vi "LVClass_Pupil AND operator.vi"(0 "Pupil A in":refnum<class "Pupil.lvclass">, 5 "Pupil B":refnum<class "Pupil.lvclass">, 11 "error in (no error)":errorcluster) -> (4 "Pupil A out":refnum<class "Pupil.lvclass">, 15 "error out":errorcluster)   [LabVIEW 2020, in "Pupil.lvclass"]
doc: "Pupil assignment.\n\n--------------------------------------------------------------------------------\n\n<B>Pupil_dstIn </B> : Pupil object.\n<B>Pupil_dstOut </B> : Pupil object.\n<B>Pupil_src </B> : Pupil object to copy.\n<B>ErrorIn </B> : Error\n<B>ErrorOut </B> : Error\n\n--------------------------------------------------------------------------------"
uses:
  Pupil.lvclass
  Pupil.lvclass/Pupil.ctl
  LVClass_Pupil Read Pupil.vi
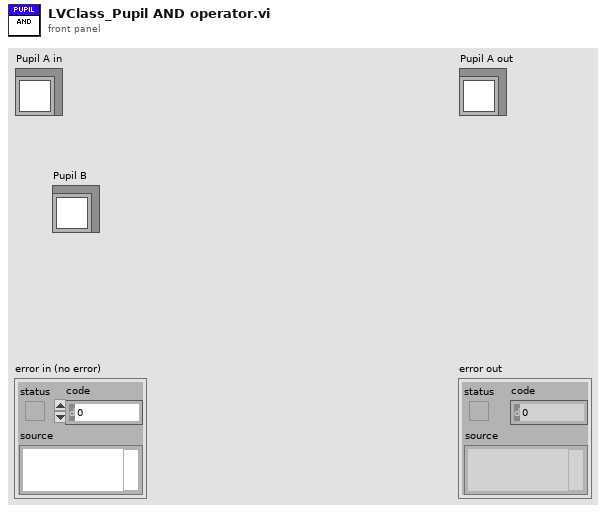
[diagram p1: front panel]
types:
  T1 = typedef "ClassID.ctl" = i64
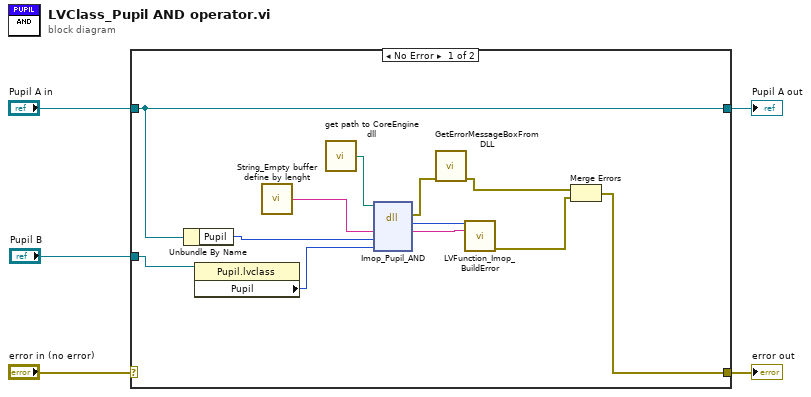
[diagram p0: block diagram]
diagram:
  n1 = case shown="No Error" "error in (no error)" {
    selector: "error in (no error)" -> [_ w19]
    tunnel: [w6 w19] -> w5
    tunnel: [w12 w18] -> w4
    tunnel: "Pupil A in" -> [w12 w18]
    tunnel: "Pupil B" -> [w10 _]
    frame No Error {
      n2 = Unbundle By Name(w12) -> ("Pupil"=w11:T1)
      n3 = property class="Pupil.lvclass"(reference=w10) -> ("Pupil"=w9:T1)  [unwired: 1 in, 2 out]
      n4 = call "String_Empty buffer define by lenght.vi"() -> ("Empty buffer"=w17:string)  [unwired: 1 in]
      n5 = call "get path to CoreEngine dll.vi"() -> ("path to wavekit library"=w14:path)  [unwired: 14 in, 1 out]
      n6 = dll-call lib="D:/soft/HASO_v3/SVN_trunk/ImOpCoreEngine4_LV2011/DLLs/c_interface_vc100.dll" fn="Imop_Pupil_AND"(path in=w14, "message"=w17, "objet"=w11, "pupil B"=w9) -> (error out=w13:errorcluster, "return type"=w15:i32, "message"=w16:string)  [unwired: 4 in, 1 out]
      n7 = call "GetErrorMessageBoxFromDLL.vi"("error IN"=w13) -> ("error OUT"=w8:errorcluster)  [unwired: 10 in]
      n8 = call "LVFunction_Imop_BuildError.vi"("code"=w15, "String to Prepend to source (\"\")"=w16) -> ("error out"=w7:errorcluster)  [unwired: 13 in]
      n9 = Merge Errors(w8, w7) -> (w6:errorcluster)
    }
    frame Error {
    }
  }
  "error out" <- w5
  "Pupil A out" <- w4
